vi "Run ExitLabVIEW.vi"   [LabVIEW 2014]
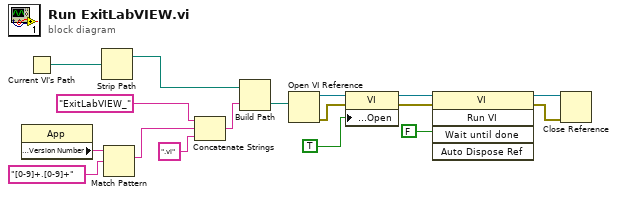
[diagram p0: block diagram]
diagram:
  n1 = property class="App"() -> ("Application:Version Number"=w3:string)  [unwired: 2 in, 2 out]
  n2 = Current VI's Path() -> (path=w16:path)
  n3 = Strip Path(path=w16) -> (stripped path=w17:path)  [unwired: 1 out]
  n4 = Match Pattern(string=w3, regular expression="[0-9]+.[0-9]+") -> (match substring=w2:string)  [unwired: 1 in, 3 out]
  n5 = Concatenate Strings("ExitLabVIEW_" ("name or relative path"), w2, ".vi" ("string")) -> (w11:string)
  n6 = Build Path(base path=w17, name or relative path=w11) -> (appended path=w15:path)
  n7 = Open VI Reference(vi path=w15) -> (vi reference=w8:refnum<vi>, error out=w7:errorcluster)  [unwired: 5 in]
  n8 = property class="VI"(reference=w8, error in=w7, "Front Panel Window:Open"=TRUE) -> (reference out=w6:refnum<vi>, error out=w5:errorcluster)
  n9 = invoke class="VI" method="Run VI"(reference=w6, error in=w5, "Wait until done"=FALSE ("Wait Until Done")) -> (reference out=w12:refnum<vi>, error out=w13:errorcluster)  [unwired: 2 in, 3 out]
  n10 = Close Reference(reference=w12, error in (no error)=w13) -> ()  [unwired: 1 out]
